vi "libssh2_sftp_mkdir.vi"(7 "mode":i32(ring) items=["LIBSSH2_SFTP_S_IRWXU"=448, "LIBSSH2_SFTP_S_IRUSR"=256, "LIBSSH2_SFTP_S_IWUSR"=128, "LIBSSH2_SFTP_S_IXUSR"=64, "LIBSSH2_SFTP_S_IRWXG"=56, "LIBSSH2_SFTP_S_IRGRP"=32, "LIBSSH2_SFTP_S_IWGRP"=16, "LIBSSH2_SFTP_S_IXGRP"=8, "LIBSSH2_SFTP_S_IRWXO"=7, "LIBSSH2_SFTP_S_IROTH"=4, "LIBSSH2_SFTP_S_IWOTH"=2, "LIBSSH2_SFTP_S_IXOTH"=1], 8 "error in (no error)":errorcluster, 10 "path":string, 11 "sftp":T1) -> (0 "error out":errorcluster)   [LabVIEW 2013, in "libssh2.lvlib"]
doc: "Create a folder on SSH server."
uses:
  libssh2.lvlib
  SFTP Refnum.ctl
  Not a SFTP Refnum.vi
  <vilib>/Utility/error.llb/Error Cluster From Error Code.vi
  Global Settings.vi
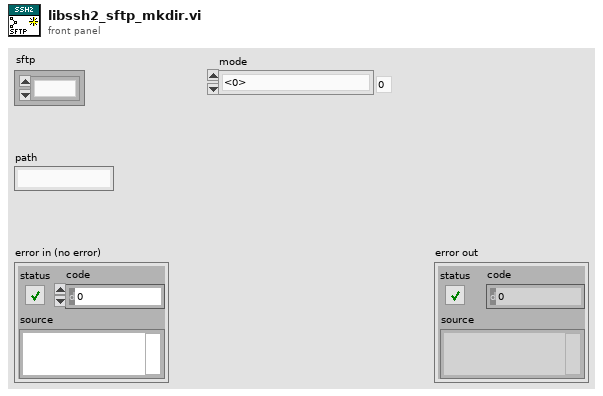
[diagram p1: front panel]
types:
  T1 = typedef "libssh2.lvlib/SFTP Refnum.ctl" = refnum<k1>
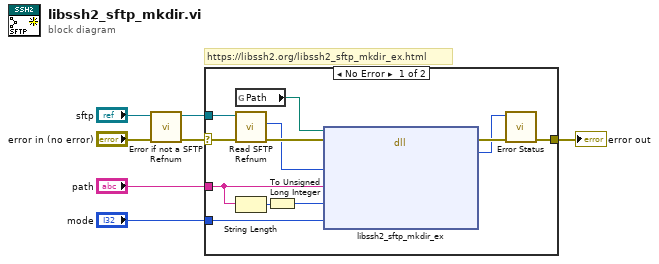
[diagram p0: block diagram]
diagram:
  # "https://libssh2.org/libssh2_sftp_mkdir_ex.html"
  n1 = call "Error if not a SFTP Refnum.vi"("error in (no error)"="error in (no error)", "sftp"="sftp") -> ("error out"=w6:errorcluster, "sftp out"=w5:T1)  [unwired: 8 in]
  n2 = case shown="No Error" w6 {
    selector: w6 -> [w18 w20]
    tunnel: w5 -> [w17 _]
    tunnel: [w13 w20] -> w4
    tunnel: "path" -> [w11 _]
    tunnel: "mode" -> [w8 _]
    frame No Error {
      n3 = global read "Global Settings.vi" "Path"() -> (w19:path)
      n4 = call "Read SFTP Refnum.vi"("error in (no error)"=w18, "sftp"=w17) -> ("error out"=w16:errorcluster, "LIBSSH2_SFTP*"=w15:u64)  [unwired: 8 in]
      n5 = String Length(string=w11) -> (length=w10:i32)
      n6 = To Unsigned Long Integer(number=w10) -> (unsigned 32bit integer=w9:u32)
      n7 = dll-call lib="?" fn="libssh2_sftp_mkdir_ex"(path in=w19, error in=w16, "sftp"=w15, "path"=w11, "path_len"=w9, "mode"=w8) -> (error out=w14:errorcluster, "return value"=w12:i32)  [unwired: 5 in, 1 out]
      n8 = call "Error Status.vi"("error in (no error)"=w14, "return value"=w12) -> ("error out"=w13:errorcluster)  [unwired: 8 in, 1 out]
    }
    frame Error {
    }
  }
  "error out" <- w4
